vi "Global_SM Write_Data Out.vi"() -> ()   [LabVIEW 2017, in "Arm.lvlib"]
uses:
  Arm.lvlib
  CLUSTER_ElbowInput.ctl
  <vilib>/Rock Robotics/WPI/ThirdParty/Phoenix-LabVIEW/Motor Controller/Controls/CTRE_Phoenix_MotorControl_ControlMode.ctl
  CLUSTER_PID.ctl
panel:
  in  "Arm_SM_Elbow_Input":T1 {"Talon Mode" items=["PercentOutput"=0, "Position"=1, "Velocity"=2, "Current"=3, "Follower"=5, "MotionProfile"=6, "MotionMagic"=7, "MotionMagicArc"=8, "MotionProfileArc"=10, "Disabled"=15]}
  # "The Names of the Data items in the Global Variable MUST describe who the Single Writer is\nNaming Convention of all Data Items is:   \nLib Name_Loop Name (SM or SEN or ACT)_Data Name\nExamples:\nDrive_ACT_X axis\nGameController_SEN_JoystickLeft\nHopper_SM_AgitatorSpeed"
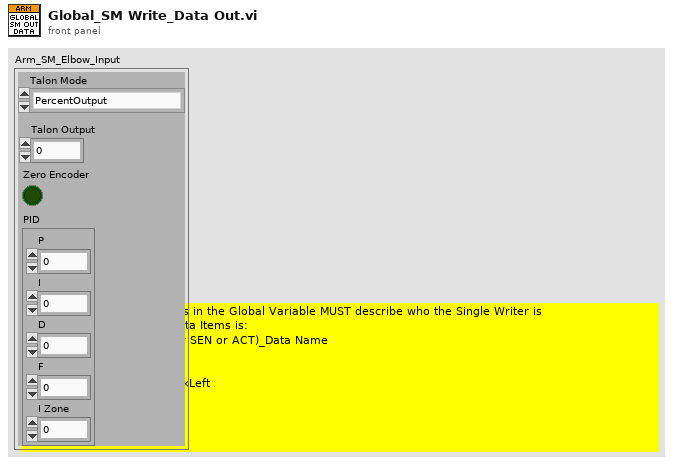
[diagram p1: front panel]
types:
  T1 = typedef "Arm.lvlib/CLUSTER_ElbowInput.ctl" = cluster{"Talon Mode":T2, "Talon Output":dbl, "Zero Encoder":bool, "PID":T3}
  T2 = typedef "CTRE_Phoenix_MotorControl_ControlMode.ctl" = u16
  T3 = typedef "Arm.lvlib/CLUSTER_PID.ctl" = cluster{"P":dbl, "I":dbl, "D":dbl, "F":dbl, "I Zone":dbl}
diagram:
